vi "REV ticks to degrees.vi"(11 "ticks":dbl) -> (3 "degrees":dbl)   [LabVIEW 2020]
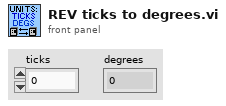
[diagram p1: front panel]
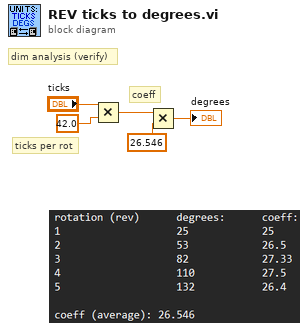
[diagram p0: block diagram]
diagram:
  # "dim analysis (verify)"
  # "coeff"
  # "ticks per rot"
  n1 = Multiply(x="ticks", y=42.0) -> (x*y=w3:dbl)
  n2 = Multiply(x=w3, y=26.546) -> (x*y=→"degrees":dbl)
